vi "CmdSet_Resp_OMAN.vi"(7 "nodeID":string, 10 "resp in":string, 11 "cmd in":string) -> (2 "resp out":string)   [LabVIEW 2016]
panel:
  in  "nodeID 2":string
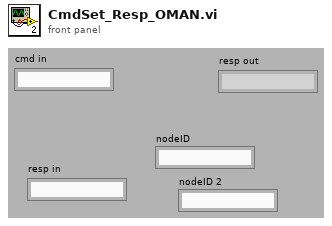
[diagram p1: front panel]
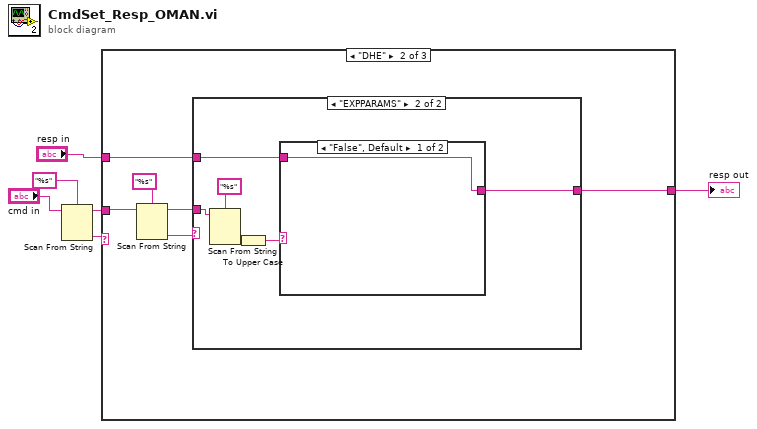
[diagram p0: block diagram]
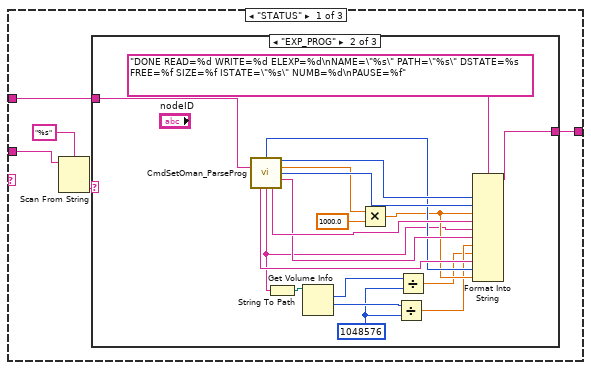
[diagram p2: hidden frame]
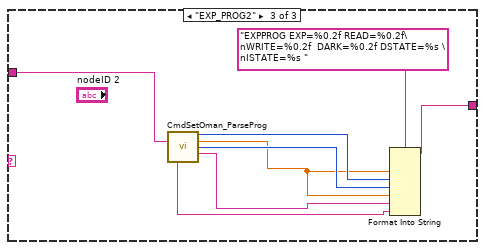
[diagram p4: hidden frame]
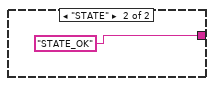
[diagram p6: hidden frame]
diagram:
  n1 = Scan From String(format string="%s", input string="cmd in") -> (remaining string=w1:string, output 1=w4:string)  [unwired: 2 in, 3 out]
  n2 = case shown="\"DHE\"" w4 {
    tunnel: "resp in" -> [w8 w42 w55]
    tunnel: [w7 w41 w55] -> w2
    tunnel: w1 -> [w11 w45 _]
    frame "STATUS" {
      n3 = Scan From String(format string="%s", input string=w11) -> (output 1=w9:string)  [unwired: 2 in, 4 out]
      n4 = case shown="\"EXP_PROG\"" w9 {
        tunnel: w8 -> [w12 w31 w39]
        tunnel: [w12 w25 w37] -> w7
        frame Default {
        }
        frame "EXP_PROG" {
          w14 = i64 1048576 ("y")
          n5 = call "CmdSetOman_ParseProg.vi"("progress"=w31) -> ("imnumber"=w21:i32, "read prog"=w29:i32, "exp prog"=w27:dbl, "write prog"=w28:i32, "detstatus"=w23:string, "imstatus"=w22:string, "imagepath"=w19:string, "imagename"=w24:string)  [unwired: 7 out]
          n6 = String To Path(string=w19) -> (path=w18:path)
          n7 = Get Volume Info(11:w18) -> (1:w17:i64, 2:w15:i64)  [unwired: 1 in, 4 out]
          n8 = Multiply(x=w27, y=1000.0) -> (x*y=w20:dbl)
          n9 = Divide(x=w17, y=w14) -> (x/y=w16:dbl)
          n10 = Divide(x=w15, y=w14) -> (x/y=w13:dbl)
          n11 = Format Into String(format string="DONE READ=%d WRITE=%d ELEXP=%d\nNAME=\"%s\" PATH=\"%s\" DSTATE=%s FREE=%f SIZE=%f ISTATE=\"%s\" NUMB=%d\nPAUSE=%f", w29, w28, w20, w24, w19, w23, w16, w13, w22, w21, w20) -> (resulting string=w25:string)  [unwired: 2 in, 1 out]
        }
        frame "EXP_PROG2" {
          n12 = call "CmdSetOman_ParseProg.vi"("progress"=w39) -> ("read prog"=w36:i32, "exp prog"=w32:dbl, "write prog"=w35:i32, "detstatus"=w34:string, "imstatus"=w33:string)  [unwired: 10 out]
          n13 = Format Into String(format string="EXPPROG EXP=%0.2f READ=%0.2f\nWRITE=%0.2f  DARK=%0.2f DSTATE=%s \nISTATE=%s ", w32, w36, w35, w32, w34, w33) -> (resulting string=w37:string)  [unwired: 2 in, 1 out]
        }
      }
    }
    frame "DHE" {
      n14 = Scan From String(format string="%s", input string=w45) -> (remaining string=w40:string, output 1=w43:string)  [unwired: 2 in, 3 out]
      n15 = case shown="\"EXPPARAMS\"" w43 {
        tunnel: w42 -> [w46 w47]
        tunnel: [w46 w52] -> w41
        tunnel: w40 -> [_ w51]
        frame Default {
        }
        frame "EXPPARAMS" {
          n16 = Scan From String(format string="%s", input string=w51) -> (output 1=w49:string)  [unwired: 2 in, 4 out]
          n17 = To Upper Case(1:w49) -> (0:w48:string)
          n18 = case shown="\"False\", Default" w48 {
            tunnel: [w53 "STATE_OK" ("resp in")] -> w52
            tunnel: w47 -> [w53 _]
            frame "False", Default {
            }
            frame "STATE" {
            }
          }
        }
      }
    }
    frame Default {
    }
  }
  "resp out" <- w2
